vi "findBox.vi"() -> ()   [LabVIEW 2017]
panel:
  out "Y_area(w*h)":dbl
  out "G_area(w*h)":dbl
  out "O_area(w*h)":dbl
  out "R_area(w*h)":dbl
  out "B_area(w*h)":dbl
  out "Yellow_Data":dbl[](array[numeric])
  out "yellow_found":bool
  out "yellow_stop":bool
  out "green_found":bool
  out "Green_Data":dbl[](array[numeric])
  out "green_stop":bool
  out "orange_stop":bool
  out "orange_found":bool
  out "Orange_Data":dbl[](array[numeric])
  out "red_found":bool
  out "Red_Data":dbl[](array[numeric])
  out "red_stop":bool
  out "blue_found":bool
  out "Blue_Data":dbl[](array[numeric])
  out "blue_stop":bool
  # "0 center x"
  # "1 center y"
  # "2 left"
  # "3 up"
  # "4 right"
  # "5 bot"
  # "6 width"
  # "7 height"
  # "8 tayang"
  # "9 area"
  # "10 convex hull area"
  # "11 img area"
  # "12 %area/img area"
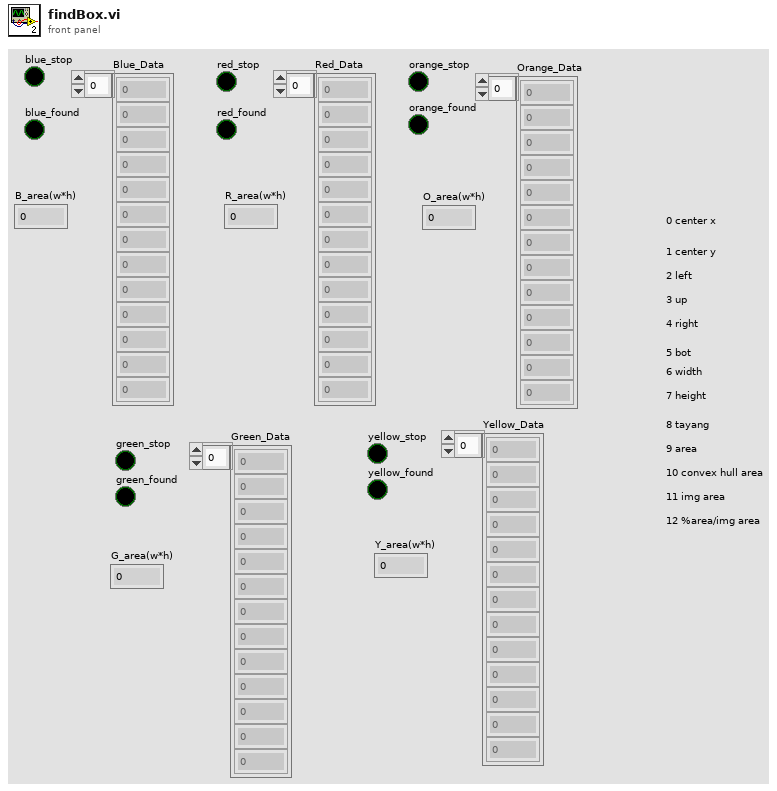
[diagram p1: front panel]
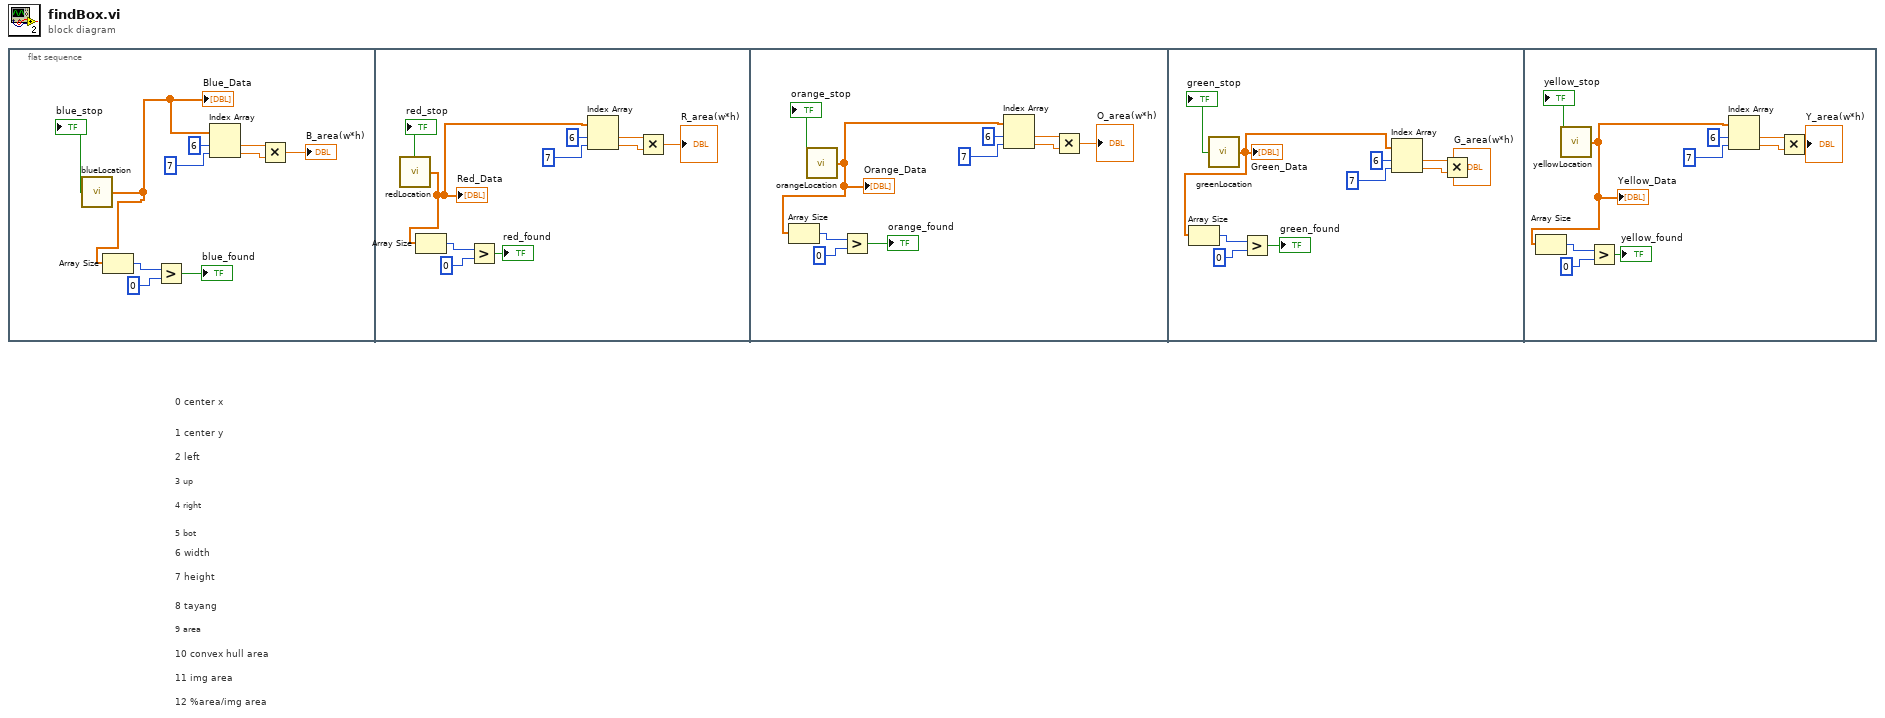
[diagram p0: block diagram]
diagram:
  # "12 %area/img area"
  # "11 img area"
  # "10 convex hull area"
  # "9 area"
  # "8 tayang"
  # "7 height"
  # "6 width"
  # "5 bot"
  # "4 right"
  # "3 up"
  # "2 left"
  # "1 center y"
  # "0 center x"
  n1 = flat-sequence {
    frame #0 {
      n2 = call "blueLocation.vi"() -> ("Blue_Data"=w6:dbl[], "blue_stop"=→"blue_stop":bool)
      "Blue_Data" <- w6
      n3 = Array Size(array=w6) -> (size(s)=w9:i32)
      n4 = Greater?(x=w9, y=0) -> (0:→"blue_found":bool)
      n5 = Index Array(array=w6, index #1=6 ("index"), index #2=7 ("index")) -> (element #1=w3:dbl, element #2=w2:dbl)
      n6 = Multiply(x=w3, y=w2) -> (x*y=→"B_area(w*h)":dbl)
    }
    frame #1 {
      n7 = call "redLocation.vi"() -> ("Red_Data"=w12:dbl[], "red_stop"=→"red_stop":bool)
      "Red_Data" <- w12
      n8 = Array Size(array=w12) -> (size(s)=w20:i32)
      n9 = Greater?(x=w20, y=0) -> (0:→"red_found":bool)
      n10 = Index Array(array=w12, index #1=6 ("index"), index #2=7 ("index")) -> (element #1=w14:dbl, element #2=w13:dbl)
      n11 = Multiply(x=w14, y=w13) -> (x*y=→"R_area(w*h)":dbl)
    }
    frame #2 {
      n12 = call "orangeLocation.vi"() -> ("Orange_Data"=w22:dbl[], "orange_stop"=→"orange_stop":bool)
      "Orange_Data" <- w22
      n13 = Array Size(array=w22) -> (size(s)=w30:i32)
      n14 = Greater?(x=w30, y=0) -> (0:→"orange_found":bool)
      n15 = Index Array(array=w22, index #1=6 ("index"), index #2=7 ("index")) -> (element #1=w24:dbl, element #2=w23:dbl)
      n16 = Multiply(x=w24, y=w23) -> (x*y=→"O_area(w*h)":dbl)
    }
    frame #3 {
      n17 = call "greenLocation.vi"() -> ("Green_Data"=w32:dbl[], "green_stop"=→"green_stop":bool)
      "Green_Data" <- w32
      n18 = Array Size(array=w32) -> (size(s)=w40:i32)
      n19 = Greater?(x=w40, y=0) -> (0:→"green_found":bool)
      n20 = Index Array(array=w32, index #1=6 ("index"), index #2=7 ("index")) -> (element #1=w34:dbl, element #2=w33:dbl)
      n21 = Multiply(x=w34, y=w33) -> (x*y=→"G_area(w*h)":dbl)
    }
    frame #4 {
      n22 = call "yellowLocation.vi"() -> ("Yellow_Data"=w42:dbl[], "yellow_stop"=→"yellow_stop":bool)
      "Yellow_Data" <- w42
      n23 = Array Size(array=w42) -> (size(s)=w50:i32)
      n24 = Greater?(x=w50, y=0) -> (0:→"yellow_found":bool)
      n25 = Index Array(array=w42, index #1=6 ("index"), index #2=7 ("index")) -> (element #1=w44:dbl, element #2=w43:dbl)
      n26 = Multiply(x=w44, y=w43) -> (x*y=→"Y_area(w*h)":dbl)
    }
  }
